vi "findAllNodesFromPath.vi"(8 "error in (no error)":errorcluster, 9 "searchElement":string, 10 "nodePath":string, 11 "xmlNode in":refnum<class "xmlNode.lvclass">) -> (0 "error out":errorcluster, 2 "arrayXmlNodes":refnum<class "xmlNode.lvclass">[](array[class]), 3 "xmlNode out":refnum<class "xmlNode.lvclass">)   [LabVIEW 2009, in "Tools.lvlib" / "xml.lvlib" / "xmlNode.lvclass"]
uses:
  xmlNode.lvclass
  XmlParser.lvclass
panel:
  out "xml":string
  out "Array":string[](array[string])
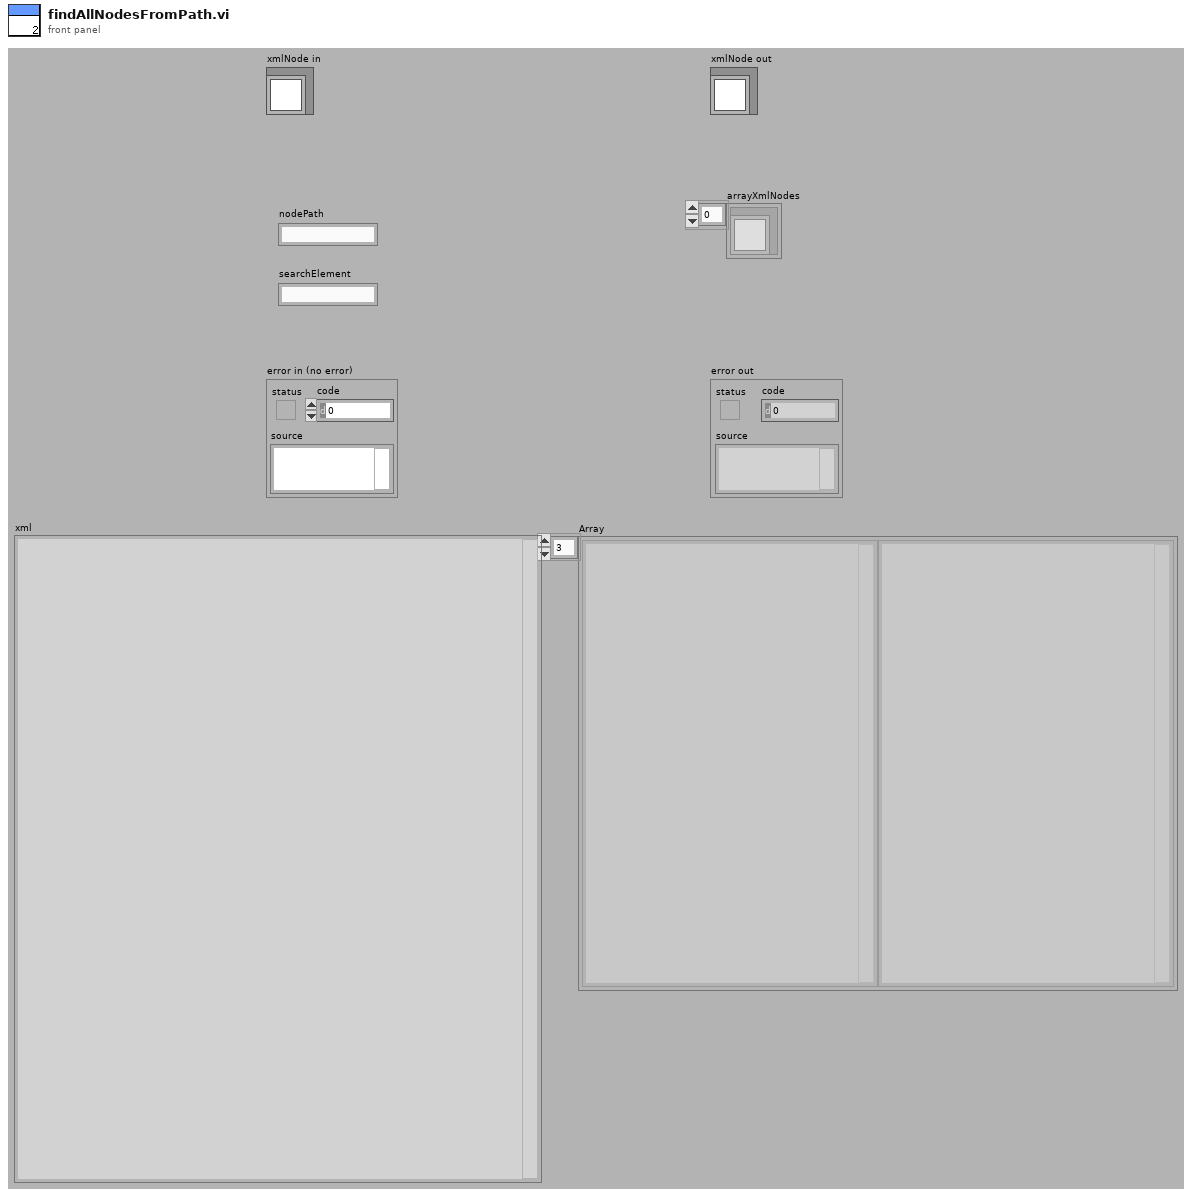
[diagram p1: front panel]
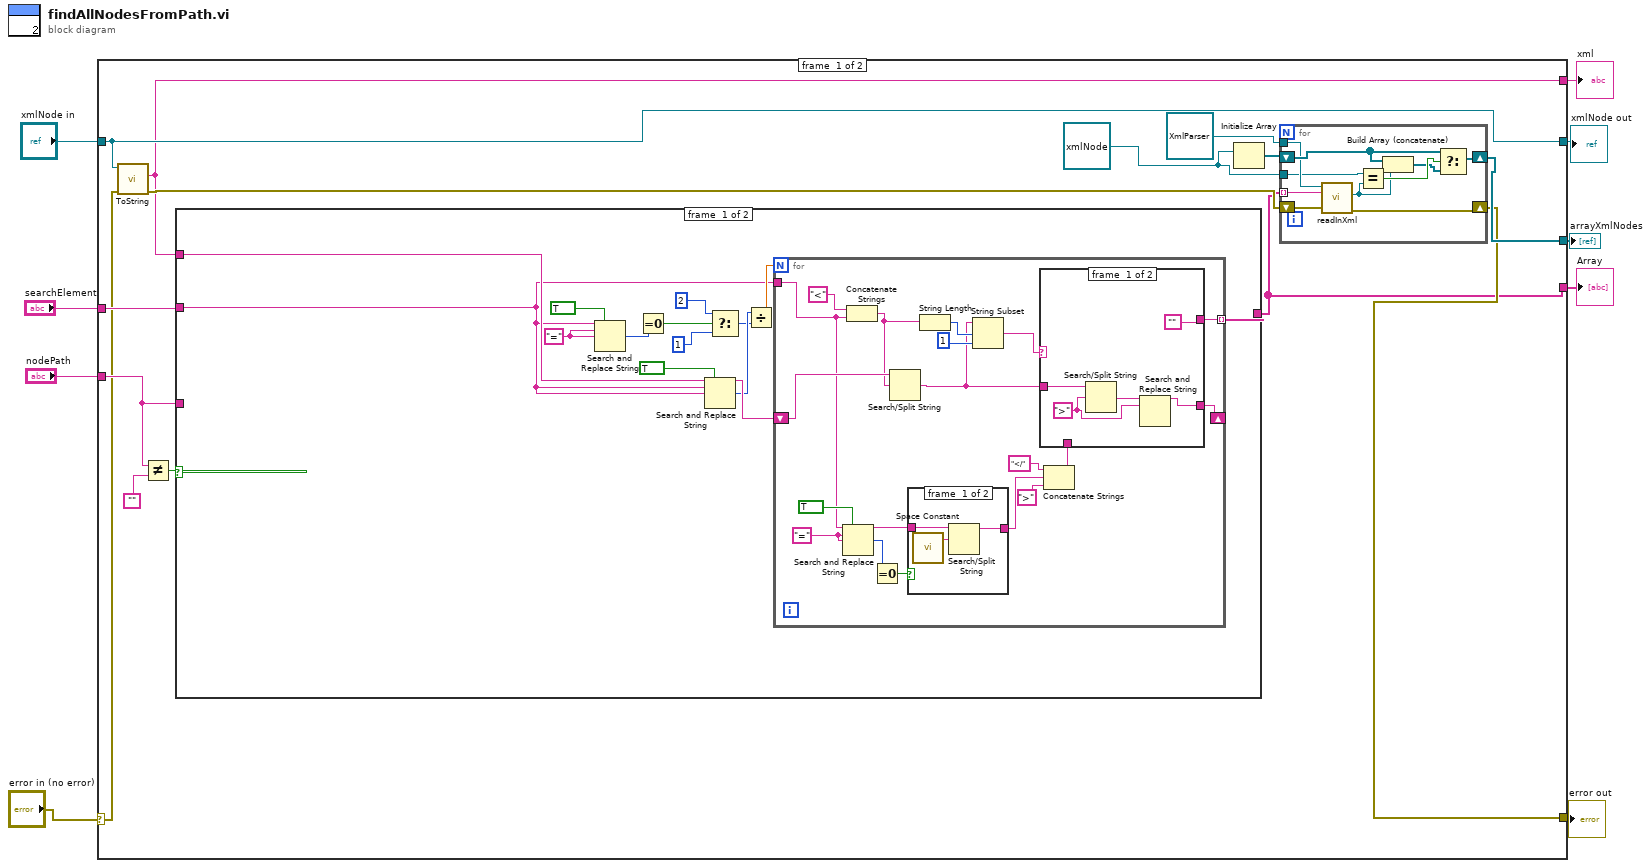
[diagram p0: block diagram]
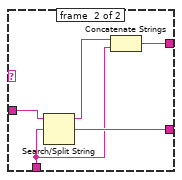
[diagram p2: hidden frame]
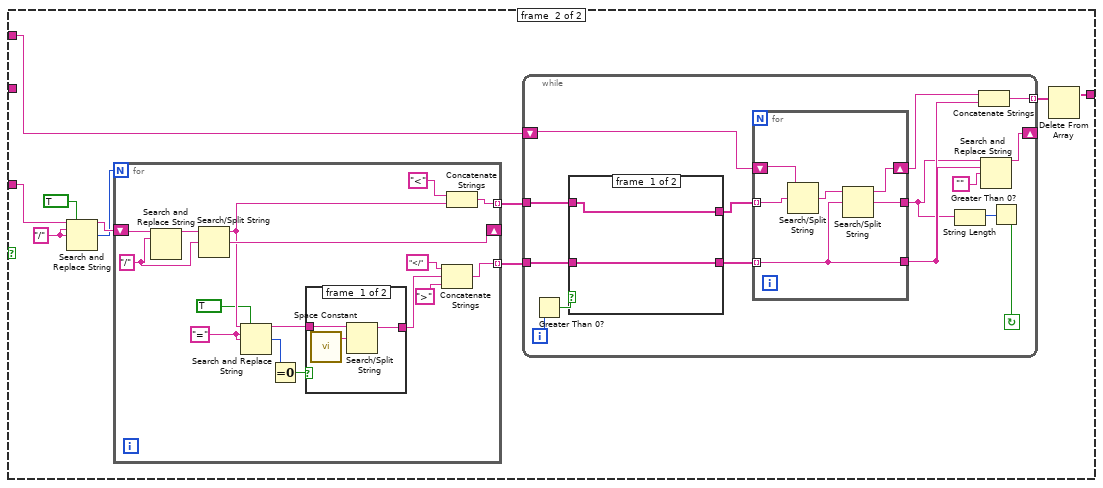
[diagram p4: hidden frame]
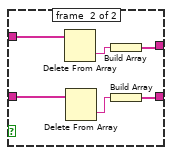
[diagram p5: hidden frame]
diagram:
  n1 = case shown="No Error" "error in (no error)" {
    selector: "error in (no error)" -> [w18 w141]
    tunnel: [w12 w141] -> w8
    tunnel: [w23 w140] -> w6
    tunnel: "xmlNode in" -> [w23 w140]
    tunnel: "nodePath" -> [w19 _]
    tunnel: "searchElement" -> [w20 _]
    tunnel: [w13 _] -> w3
    tunnel: [w11 _] -> w2
    tunnel: [w10 _] -> w1
    frame #0 {
      w14 = refnum<class "xmlNode.lvclass"> refnum ("Tools.lvlib:xml.lvlib:xmlNode.lvclass")
      n2 = call-dynamic "ToString.vi"("error in (no error)"=w18, "xmlNode in"=w23) -> ("error out"=w16:errorcluster, "xml"=w10:string)  [unwired: 7 in, 1 out]
      n3 = Not Equal?(x=w19, y="") -> (x != y?=w21:bool)
      n4 = case shown="False" w21 {
        tunnel: [w36 w83] -> w11
        tunnel: w10 -> [w35 w82]
        tunnel: w19 -> [_ w81]
        tunnel: w20 -> [w34 _]
        frame #0 {
          w43 = "="
          n5 = Search and Replace String(replace all?=TRUE, input string=w34, search string=w43, replace string=w43) -> (number of replacements=w42:i32)  [unwired: 4 in, 3 out]
          n6 = Equal To 0?(x=w42) -> (x = 0?=w37:bool)
          n7 = Search and Replace String(replace all?=TRUE, input string=w35, search string=w34, replace string=w34) -> (result string=w46:string, number of replacements=w44:i32)  [unwired: 4 in, 2 out]
          n8 = Select(t=2, s=w37, f=1) -> (s? t:f=w40:i32)
          n9 = Divide(x=w44, y=w40) -> (x/y=w45:dbl)
          n10 = for {
            N: w45 -> [_]
            tunnel: w34 -> [w56]
            shift-right: [w55] -> _
            shift-left: w46 -> [w66]
            tunnel: [w54] -> w36 mode=indexing
            w62 = "="
            n11 = Search and Replace String(replace all?=TRUE, input string=w56, search string=w62, replace string=w62) -> (result string=w59:string, number of replacements=w61:i32)  [unwired: 4 in, 2 out]
            n12 = Concatenate Strings("<", w56) -> (w50:string)
            n13 = Equal To 0?(x=w61) -> (x = 0?=w60:bool)
            n14 = Search/Split String(string=w66, search string/char (-)=w50) -> (match + rest of string=w49:string)  [unwired: 1 in, 2 out]
            n15 = case shown="True" w60 {
              tunnel: w59 -> [w79 w80]
              tunnel: [w77 w80] -> w58
              frame #0 {
                n16 = call <vilib>:"Space Constant.vi"() -> ("String"=w78:string)
                n17 = Search/Split String(string=w79, search string/char (-)=w78) -> (substring before match=w77:string)  [unwired: 1 in, 2 out]
              }
              frame #1 {
              }
            }
            n18 = String Length(string=w50) -> (length=w51:i32)
            n19 = String Subset(string=w49, offset (0)=w51, length (rest)=1) -> (substring=w48:string)
            n20 = Concatenate Strings("</", w58, ">") -> (w53:string)
            n21 = case shown="\"False\", Default" w48 {
              tunnel: [w68 w76] -> w55
              tunnel: w49 -> [w71 w75]
              tunnel: ["" w74] -> w54
              tunnel: w53 -> [_ w72]
              frame #0 {
                w69 = ">"
                n22 = Search/Split String(string=w71, search string/char (-)=w69) -> (match + rest of string=w70:string)  [unwired: 1 in, 2 out]
                n23 = Search and Replace String(input string=w70, search string=w69) -> (result string=w68:string)  [unwired: 6 in, 3 out]
              }
              frame #1 {
                n24 = Search/Split String(string=w75, search string/char (-)=w72) -> (substring before match=w73:string, match + rest of string=w76:string)  [unwired: 1 in, 1 out]
                n25 = Concatenate Strings(w73, w72) -> (w74:string)
              }
            }
          }
        }
        frame #1 {
          w88 = "/"
          n26 = Search and Replace String(replace all?=TRUE, input string=w81, search string=w88, replace string=w88) -> (result string=w90:string, number of replacements=w89:i32)  [unwired: 4 in, 2 out]
          n27 = for {
            N: w89 -> [_]
            tunnel: [w129] -> w87 mode=indexing
            tunnel: [w128] -> w86 mode=indexing
            shift-right: [w127] -> _
            shift-left: w90 -> [w135]
            w125 = "="
            w134 = "/"
            n28 = Search and Replace String(input string=w135, search string=w134) -> (result string=w133:string)  [unwired: 6 in, 3 out]
            n29 = Search/Split String(string=w133, search string/char (-)=w134) -> (substring before match=w126:string, match + rest of string=w127:string)  [unwired: 1 in, 1 out]
            n30 = Search and Replace String(replace all?=TRUE, input string=w126, search string=w125, replace string=w125) -> (result string=w122:string, number of replacements=w124:i32)  [unwired: 4 in, 2 out]
            n31 = Equal To 0?(x=w124) -> (x = 0?=w123:bool)
            n32 = case shown="False" w123 {
              tunnel: w122 -> [w138 w139]
              tunnel: [w136 w139] -> w121
              frame #0 {
                n33 = call <vilib>:"Space Constant.vi"() -> ("String"=w137:string)
                n34 = Search/Split String(string=w138, search string/char (-)=w137) -> (substring before match=w136:string)  [unwired: 1 in, 2 out]
              }
              frame #1 {
              }
            }
            n35 = Concatenate Strings("</", w121, ">") -> (w128:string)
            n36 = Concatenate Strings("<", w126) -> (w129:string)
          }
          n37 = while {
            tunnel: w87 -> [w101]
            tunnel: w86 -> [w100]
            shift-right: [w102] -> _
            shift-left: w82 -> [w91]
            tunnel: [w105] -> w84 mode=indexing
            i -> [w93]
            stop <- w92 continue-if-true
            n38 = Greater Than 0?(x=w93) -> (x > 0?=w99:bool)
            n39 = case shown="True" w99 {
              tunnel: w101 -> [w107 w112]
              tunnel: w100 -> [w106 w113]
              tunnel: [w107 w110] -> w96
              tunnel: [w106 w108] -> w95
              frame #0 {
              }
              frame #1 {
                n40 = Delete From Array(array=w112) -> (deleted portion=w111:string)  [unwired: 2 in, 1 out]
                n41 = Delete From Array(array=w113) -> (deleted portion=w109:string)  [unwired: 2 in, 1 out]
                n42 = Build Array(w111) -> (w110:string[])
                n43 = Build Array(w109) -> (w108:string[])
              }
            }
            n44 = for {
              tunnel: w96 -> [w115] mode=indexing
              tunnel: w95 -> [w114] mode=indexing
              shift-right: [w117] -> w94
              shift-left: w91 -> [w119]
              tunnel: [w114] -> w98
              tunnel: [w116] -> w97
              n45 = Search/Split String(string=w119, search string/char (-)=w115) -> (match + rest of string=w118:string)  [unwired: 1 in, 2 out]
              n46 = Search/Split String(string=w118, search string/char (-)=w114) -> (substring before match=w117:string, match + rest of string=w116:string)  [unwired: 1 in, 1 out]
            }
            n47 = String Length(string=w97) -> (length=w104:i32)
            n48 = Concatenate Strings(w94, w98) -> (w105:string)
            n49 = Search and Replace String(input string=w97, search string=w98, replace string="") -> (result string=w102:string)  [unwired: 5 in, 3 out]
            n50 = Greater Than 0?(x=w104) -> (x > 0?=w92:bool)
          }
          n51 = Delete From Array(array=w84) -> (array with subset deleted=w83:string[])  [unwired: 2 in, 1 out]
        }
      }
      n52 = Initialize Array(w14) -> (w15:refnum<class "xmlNode.lvclass">[])  [unwired: 1 in]
      n53 = for {
        tunnel: w11 -> [w31] mode=indexing
        shift-right: [w32] -> w12
        shift-left: w16 -> [w33]
        shift-right: [w28] -> w13
        shift-left: w15 -> [w30]
        tunnel: refnum<class "XmlParser.lvclass"> refnum ("Tools.lvlib:XmlParser.lvclass") -> [w27]
        tunnel: w14 -> [w26]
        n54 = call "readInXml.vi"("error in (no error)"=w33, "xmlString"=w31, "XmlParser in"=w27) -> ("error out"=w32:errorcluster, "xmlNode"=w24:refnum<class "xmlNode.lvclass">)  [unwired: 6 in, 1 out]
        n55 = Equal?(x=w26, y=w24) -> (x = y?=w29:bool)
        n56 = Build Array (concatenate)(w30, w24) -> (w25:refnum<class "xmlNode.lvclass">[])
        n57 = Select(t=w30, s=w29, f=w25) -> (s? t:f=w28:refnum<class "xmlNode.lvclass">[])
      }
    }
    frame #1 {
    }
  }
  "error out" <- w8
  "xmlNode out" <- w6
  "arrayXmlNodes" <- w3
  "Array" <- w2
  "xml" <- w1
